vi "post_scan.vi"(7 "override":bool, 8 "error in (no error)":errorcluster, 11 "VISA IN":refnum<visa-resource-name>="COM9") -> (0 "error out":errorcluster)   [LabVIEW 2017, in "radiant.lvlib"]
uses:
  radiant.lvlib
panel:
  out "VISA resource out":refnum<visa-resource-name>="COM9"
  in  "VISA (default)":refnum<visa-resource-name>="COM9"
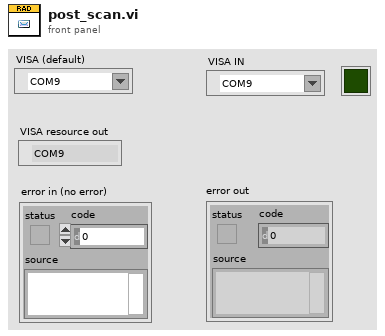
[diagram p1: front panel]
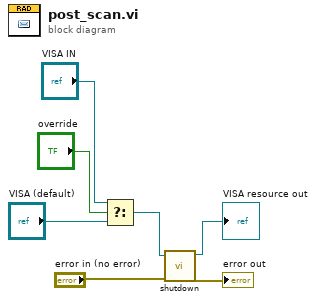
[diagram p0: block diagram]
diagram:
  n1 = Select(t="VISA IN", s="override", f="VISA (default)") -> (s? t:f=w4:refnum<visa-resource-name>)
  n2 = call "shutdown.vi"("error in (no error)"="error in (no error)", "VISA resource name"=w4) -> ("error out"=→"error out":errorcluster, "VISA resource name out"=→"VISA resource out":refnum<visa-resource-name>)  [unwired: 7 in, 1 out]
